vi "filter.vi"(8 "debug":bool, 9 "conf.valid":bool, 10 "conf":u64, 11 "reset":bool) -> (1 "Ready.for.OrderBook.Command.Input":bool, 2 "Ready.for.Configuration.Input":bool)   [LabVIEW 2022 SP3]
uses:
  filter.states.ctl
  filter.data.ctl
  filter.debug.ctl
  filter.debug.slot.ctl
  filter.data.scratch.ctl
  arty/orderbook/orderbook.command.ctl
  arty/orderbook/orderbook.command.type.ctl
  filter.memory.command.ctl
  ticker.slot.ctl
  order.slot.ctl
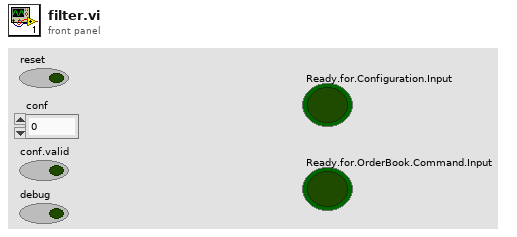
[diagram p1: front panel]
types:
  T1 = typedef "filter.data.ctl" = cluster{"filter.state":T2, "Debug":T3, "number.of.tickers":u32, "number.of.orders":u32, "filter.saved.state":T2, "Scratch":T5, "OrderBook.Command":T6, "Send.Command":bool, "memory.command":T8}
  T2 = typedef "filter.states.ctl" = enum16{"Noop", "Reset", "Debug", "Configuration", "Wait.for.Command", "Filter.Add", "Filter.Other", "Insert.Order", "Delete Order"}
  T3 = typedef "filter.debug.ctl" = cluster{"Write.to.Debug":bool, "debug.slot":T4}
  T4 = typedef "filter.debug.slot.ctl" = cluster{"Ticker":u64, "OrderId":u64}
  T5 = typedef "filter.data.scratch.ctl" = cluster{"I":u32, "N":u32, "Mode":u32, "OrderId":u64, "First Call?":bool, "Just Write":bool}
  T6 = typedef "orderbook.command.ctl" = cluster{"OrderBook Command.Type":T7, "Side (U8)":u8, "Order Id (U64)":u64, "Quantity (U32)":u32, "Symbol (U64)":u64, "Price (U64)":u64, "Executed Quantity (U32)":u32, "Canceled Quantity (U32)":u32, "Remaining Quantity (U32)":u32, "Seconds (U64)":u64, "Nanoseconds (U64)":u64}
  T7 = typedef "orderbook.command.type.ctl" = enum16{"Time", "AddOrder", "OrderExecuted", "OrderExecutedAtPrice", "ReduceSize", "ModifyOrder", "DeleteOrder", "Get.All.Orders", "Get.Top"}
  T8 = typedef "filter.memory.command.ctl" = cluster{"ticker.slot.value":T9, "order.slot.value":T10, "Write Ticker\nAddress":u32, "Write Ticker\nRequest":bool, "Read Ticker\nRequest":bool, "Read Ticker\nAddress":u32, "Read Ticker Valid":bool, "Write Order\nAddress":u32, "Write Order\nRequest":bool, "Read Order\nRequest":bool, "Read Order\nAddress":u32, "Read Order Valid":bool}
  T9 = typedef "ticker.slot.ctl" = cluster{"Symbol":u64}
  T10 = typedef "order.slot.ctl" = cluster{"OrderId":u64, "Quantity":u64}
  T11 = cluster{"reset":bool, "conf":u64, "conf.valid":bool, "debug":bool}
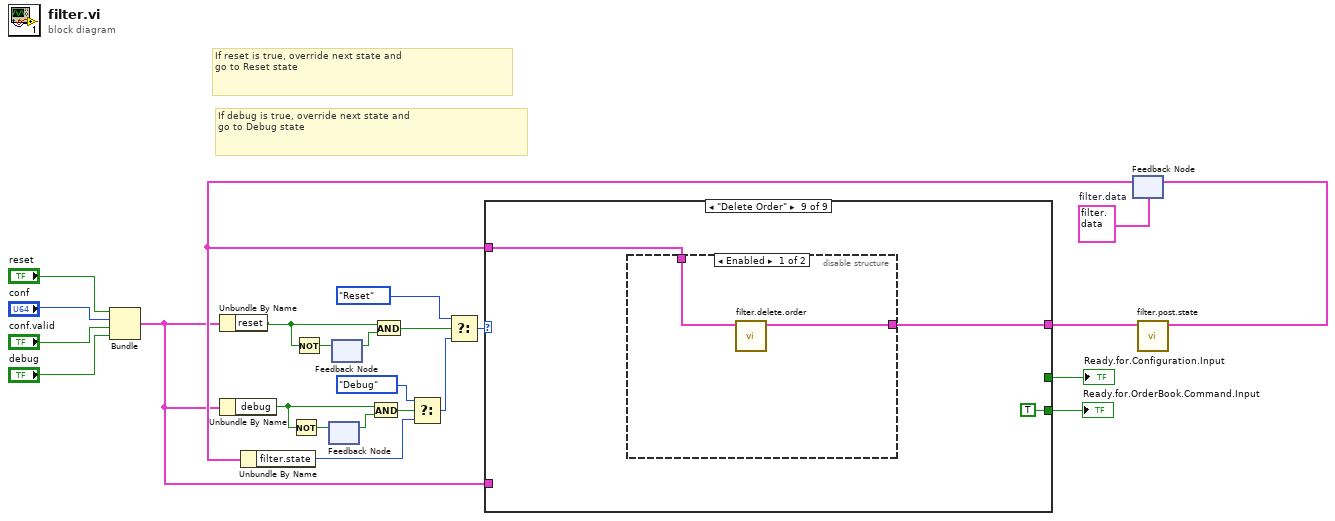
[diagram p0: block diagram]
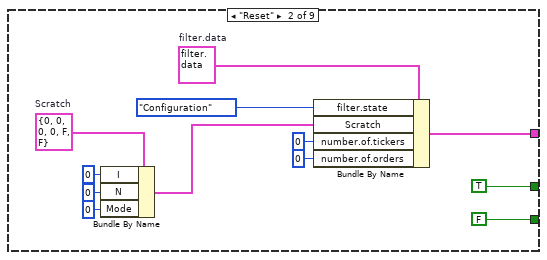
[diagram p3: hidden frame]
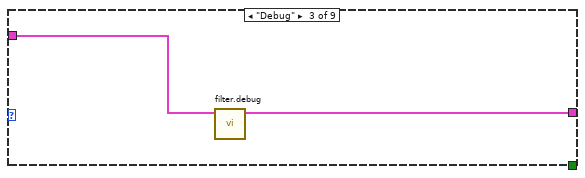
[diagram p4: hidden frame]
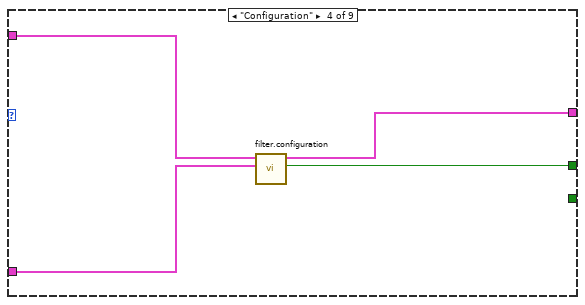
[diagram p5: hidden frame]
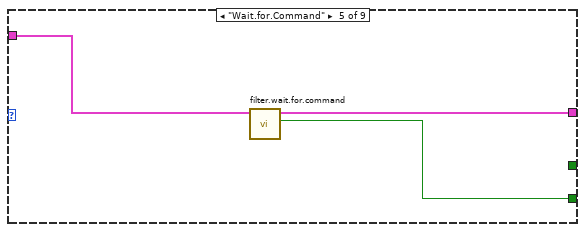
[diagram p6: hidden frame]
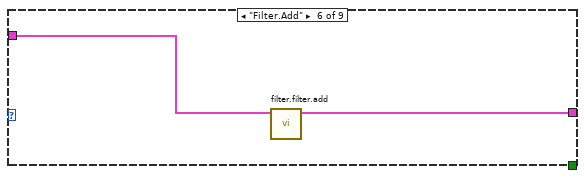
[diagram p7: hidden frame]
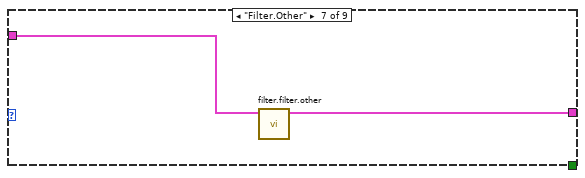
[diagram p8: hidden frame]
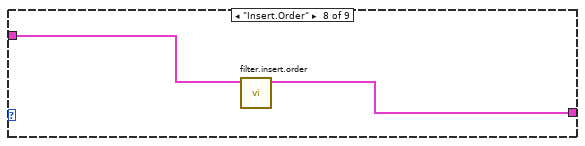
[diagram p9: hidden frame]
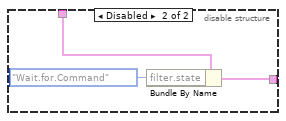
[diagram p10: hidden frame]
diagram:
  w9 = T1 {"filter.state"=enum."Noop", "Debug"={"Write.to.Debug"=FALSE, "debug.slot"={"Ticker"=0, "OrderId"=0}}, "number.of.tickers"=0, "number.of.orders"=0, "filter.saved.state"=enum."Noop", "Scratch"={"I"=0, "N"=0, "Mode"=0, "OrderId"=0, "First Call?"=FALSE, "Just Write"=FALSE}, "OrderBook.Command"={"OrderBook Command.Type"=enum."Time", "Side (U8)"=0, "Order Id (U64)"=0, "Quantity (U32)"=0, "Symbol (U64)"=0, "Price (U64)"=0, "Executed Quantity (U32)"=0, "Canceled Quantity (U32)"=0, "Remaining Quantity (U32)"=0, "Seconds (U64)"=0, "Nanoseconds (U64)"=0}, "Send.Command"=FALSE, "memory.command"={"ticker.slot.value"={"Symbol"=0}, "order.slot.value"={"OrderId"=0, "Quantity"=0}, "Write Ticker\nAddress"=0, "Write Ticker\nRequest"=FALSE, "Read Ticker\nRequest"=FALSE, "Read Ticker\nAddress"=0, "Read Ticker Valid"=FALSE, "Write Order\nAddress"=0, "Write Order\nRequest"=FALSE, "Read Order\nRequest"=FALSE, "Read Order\nAddress"=0, "Read Order Valid"=FALSE}}  # filter.data
  # "If debug is true, override next state and \ngo to Debug state"
  # "If reset is true, override next state and \ngo to Reset state"
  n1 = Bundle("reset"="reset", "conf"="conf", "conf.valid"="conf.valid", "debug"="debug") -> (w3:T11)  [unwired: 1 in]
  n2 = Unbundle By Name(w3) -> ("reset"=w18:bool)
  n3 = Unbundle By Name(w3) -> ("debug"=w15:bool)
  n4 = Not(x=w15) -> (.not. x?=w17:bool)
  n5 = Not(x=w18) -> (.not. x?=w20:bool)
  n6 = feedback #1() -> (w16:bool)  [unwired: 1 in]
  n7 = feedback-in #1(w17) -> ()
  n8 = feedback #2() -> (w19:bool)  [unwired: 1 in]
  n9 = feedback-in #2(w20) -> ()
  n10 = And(x=w15, y=w16) -> (x .and. y?=w12:bool)
  n11 = And(x=w18, y=w19) -> (x .and. y?=w13:bool)
  n12 = feedback #3(w9) -> (w6:T1)
  n13 = Unbundle By Name(w6) -> ("filter.state"=w8:T2)
  n14 = Select(t=filter.states."Debug" ("filter.states"), s=w12, f=w8) -> (s? t:f=w10:T2)
  n15 = Select(t=filter.states."Reset" ("filter.states"), s=w13, f=w10) -> (s? t:f=w7:T2)
  n16 = case shown="\"Delete Order\"" w7 {
    tunnel: [w25 w36 w39 w43 w44 w48 w49 w51 w53] -> w1
    tunnel: w6 -> [w25 _ w38 w41 w46 w47 w50 w52 w54]
    tunnel: [_ TRUE _ w40 _ _ _ _ _] -> w5
    tunnel: [_ FALSE _ _ w45 _ _ _ TRUE ("Ready.for.OrderBook.Command.Input")] -> w4
    tunnel: w3 -> [_ _ _ w42 _ _ _ _ _]
    frame "Noop", Default {
    }
    frame "Reset" {
      w32 = T5 {"I"=0, "N"=0, "Mode"=0, "OrderId"=0, "First Call?"=FALSE, "Just Write"=FALSE}  # Scratch
      w37 = T1 {"filter.state"=enum."Noop", "Debug"={"Write.to.Debug"=FALSE, "debug.slot"={"Ticker"=0, "OrderId"=0}}, "number.of.tickers"=0, "number.of.orders"=0, "filter.saved.state"=enum."Noop", "Scratch"={"I"=0, "N"=0, "Mode"=0, "OrderId"=0, "First Call?"=FALSE, "Just Write"=FALSE}, "OrderBook.Command"={"OrderBook Command.Type"=enum."Time", "Side (U8)"=0, "Order Id (U64)"=0, "Quantity (U32)"=0, "Symbol (U64)"=0, "Price (U64)"=0, "Executed Quantity (U32)"=0, "Canceled Quantity (U32)"=0, "Remaining Quantity (U32)"=0, "Seconds (U64)"=0, "Nanoseconds (U64)"=0}, "Send.Command"=FALSE, "memory.command"={"ticker.slot.value"={"Symbol"=0}, "order.slot.value"={"OrderId"=0, "Quantity"=0}, "Write Ticker\nAddress"=0, "Write Ticker\nRequest"=FALSE, "Read Ticker\nRequest"=FALSE, "Read Ticker\nAddress"=0, "Read Ticker Valid"=FALSE, "Write Order\nAddress"=0, "Write Order\nRequest"=FALSE, "Read Order\nRequest"=FALSE, "Read Order\nAddress"=0, "Read Order Valid"=FALSE}}  # filter.data
      n17 = Bundle By Name(cluster=w32, "I"=u32 0, "N"=u32 0, "Mode"=u32 0) -> (w31:T5)
      n18 = Bundle By Name(cluster=w37, "filter.state"=filter.states."Configuration", "Scratch"=w31, "number.of.tickers"=u32 0, "number.of.orders"=u32 0) -> (w36:T1)
    }
    frame "Debug" {
      n19 = call "filter.debug.vi"("filter.data in"=w38) -> ("filter.data out"=w39:T1)  [unwired: 10 in]
    }
    frame "Configuration" {
      n20 = call "filter.configuration.vi"("Cluster"=w42, "filter.data in"=w41) -> ("Boolean"=w40:bool, "filter.data out"=w43:T1)  [unwired: 8 in]
    }
    frame "Wait.for.Command" {
      n21 = call "filter.wait.for.command.vi"("filter.data in"=w46) -> ("Ready.for.OrderBook.Command.Input"=w45:bool, "filter.data out"=w44:T1)  [unwired: 9 in]
    }
    frame "Filter.Add" {
      n22 = call "filter.filter.add.vi"("filter.data in"=w47) -> ("filter.data out"=w48:T1)  [unwired: 10 in]
    }
    frame "Filter.Other" {
      n23 = call "filter.filter.other.vi"("filter.data in"=w50) -> ("filter.data out"=w49:T1)  [unwired: 10 in]
    }
    frame "Insert.Order" {
      n24 = call "filter.insert.order.vi"("filter.data in"=w52) -> ("filter.data out"=w51:T1)  [unwired: 10 in]
    }
    frame "Delete Order" {
      n25 = disable-structure shown="Enabled" {
        disable-tunnel: w54 -> [w57 w60]
        disable-tunnel: [w56 w59] -> w53
        frame Enabled {
          n26 = call "filter.delete.order.vi"("filter.data in"=w57) -> ("filter.data out"=w56:T1)  [unwired: 10 in]
        }
        frame Disabled {
          n27 = Bundle By Name(cluster=w60, "filter.state"=filter.states."Wait.for.Command") -> (w59:T1)
        }
      }
    }
  }
  "Ready.for.OrderBook.Command.Input" <- w4
  "Ready.for.Configuration.Input" <- w5
  n28 = call "filter.post.state.vi"("filter.data in"=w1) -> ("filter.data out 2"=w2:T1)  [unwired: 10 in]
  n29 = feedback-in #3(w2) -> ()
